vi "vision_webcam_V1_host.vi"() -> ()   [LabVIEW 2017]
uses:
  <vilib>/userdefined/High Color/IMAQdx.ctl
  <vilib>/vision/driver/NI_Vision_Acquisition_Software.lvlib
panel:
  in  "Session In":T1="cam0"
  in  "stop":bool
  out "Webcam":T2(plugin-control)
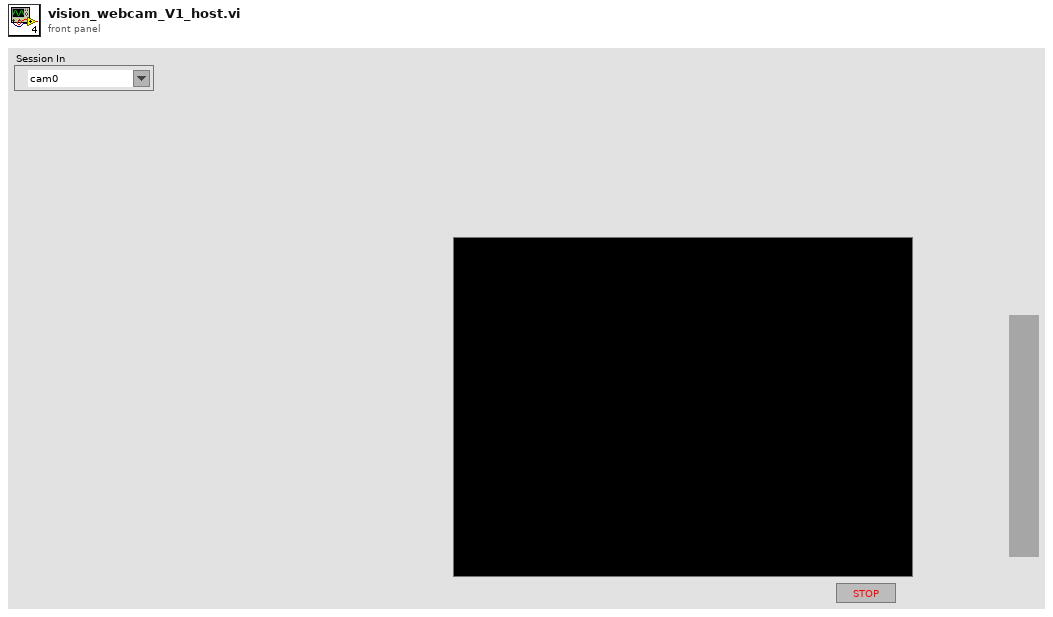
[diagram p1: front panel]
types:
  T1 = typedef "IMAQdx.ctl" = refnum<k21>
  T2 = typedef "IMAQ Image.ctl" = refnum<image>
  T3 = typedef "Image Type" = u32
  T4 = typedef "IMAQ AVI2 Refnum.ctl" = refnum<k20>
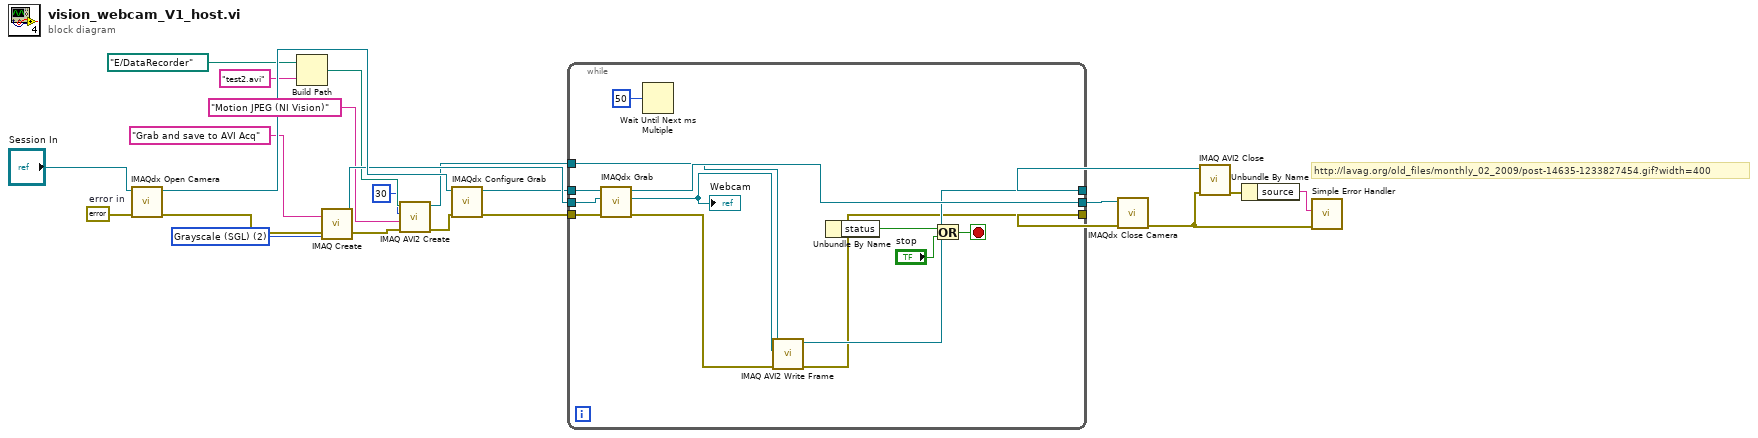
[diagram p0: block diagram]
diagram:
  w6 = T3 2 items=["Grayscale (U8)", "Grayscale (I16)", "Grayscale (SGL)", "Complex (CSG)", "RGB (U32)", "HSL (U32)", "RGB (U64)", "Grayscale (U16)"] ("Image Type")
  w17 = errorcluster {"status"=FALSE, "code"=0, "source"=""}  # error in
  # "http://lavag.org/old_files/monthly_02_2009/post-14635-1233827454.gif?width=400"
  n1 = call <vilib>:"IMAQdx Open Camera.vi"("error in"=w17, "Session In"="Session In") -> ("error out"=w5:errorcluster, "Session Out"=w23:T1)  [unwired: 8 in]
  n2 = Build Path(base path=path "E:/DataRecorder" ("AVI Path"), name or relative path="test2.avi") -> (appended path=w12:path)
  n3 = call "IMAQ Create"("Image Name"="Grab and save to AVI Acq", "Image Type"=w6, "error in (no error)"=w5) -> ("New Image"=w20:T2, "error out"=w4:errorcluster)  [unwired: 2 in]
  n4 = call "IMAQ AVI2 Create"("error in (no error)"=w4, "Codec"="Motion JPEG (NI Vision)", "Frames Per Second"=u32 30, "AVI Path"=w12) -> ("error out"=w3:errorcluster, "AVI Refnum"=w10:T4)  [unwired: 6 in]
  n5 = call <vilib>:"IMAQdx Configure Grab.vi"("error in"=w3, "Session In"=w23) -> ("error out"=w21:errorcluster, "Session Out"=w2:T1)  [unwired: 8 in]
  n6 = while {
    tunnel: w21 -> [w36]
    tunnel: w2 -> [w35]
    tunnel: w20 -> [w34]
    tunnel: [w28] -> w19
    tunnel: [w33] -> w18
    tunnel: w10 -> [w31]
    tunnel: [w30] -> w7
    stop <- w25 stop-if-true
    n7 = call <vilib>:"IMAQdx Grab.vi"("error in"=w36, "Image In"=w34, "Session In"=w35) -> ("error out"=w29:errorcluster, "Image Out"=w24:T2, "Session Out"=w33:T1)  [unwired: 5 in, 1 out]
    "Webcam" <- w24
    n8 = Wait Until Next ms Multiple(millisecond multiple=u32 50 ("milliseconds to wait")) -> ()  [unwired: 1 out]
    n9 = call "IMAQ AVI2 Write Frame"("error in (no error)"=w29, "Image"=w24, "AVI Refnum"=w31) -> ("error out"=w28:errorcluster, "AVI Refnum (duplicate)"=w30:T4)  [unwired: 6 in, 1 out]
    n10 = Unbundle By Name(w28) -> ("status"=w27:bool)
    n11 = Or(x=w27, y="stop") -> (x .or. y?=w25:bool)
  }
  n12 = call <vilib>:"IMAQdx Close Camera.vi"("error in"=w19, "Session In"=w18) -> ("error out"=w9:errorcluster)  [unwired: 9 in]
  n13 = call "IMAQ AVI2 Close"("error in (no error)"=w9, "AVI Refnum"=w7) -> ("error out"=w8:errorcluster)  [unwired: 9 in]
  n14 = Unbundle By Name(w8) -> ("source"=w15:string)
  n15 = call <vilib>:"Simple Error Handler.vi"("error source (\" \")"=w15, "error in (no error)"=w9) -> ()  [unwired: 3 in, 5 out]
